vi "Open_Close.vi"(0 "VI_Reference_In":refnum<vi>, 11 "Error_In":errorcluster, 13 "Open/Close":T1=enum."Close") -> (4 "VI_Reference_Out":refnum<vi>, 15 "Error_Out":errorcluster)   [LabVIEW 2021]
doc: "Used to open and close the VI"
uses:
  Controls/Open_Close.ctl
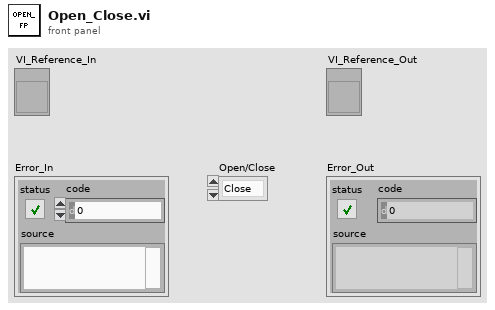
[diagram p1: front panel]
types:
  T1 = typedef "Open_Close.ctl" = enum16{"Open", "Close"}
  T2 = enum32{"Invalid", "Standard", "Closed", "Hidden", "Minimized", "Maximized"}
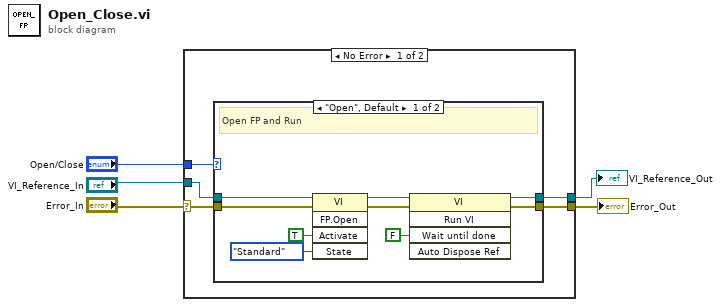
[diagram p0: block diagram]
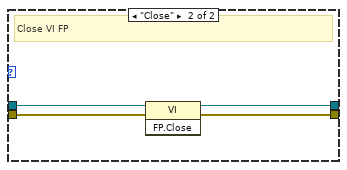
[diagram p2: hidden frame]
diagram:
  n1 = case shown="No Error" "Error_In" {
    selector: "Error_In" -> [w10 w25]
    tunnel: [w9 w25] -> w1
    tunnel: "Open/Close" -> [w8 _]
    tunnel: "VI_Reference_In" -> [w6 w24]
    tunnel: [w7 w24] -> w4
    frame No Error {
      n2 = case shown="\"Open\", Default" w8 {
        tunnel: w10 -> [w19 w22]
        tunnel: [w18 w23] -> w9
        tunnel: w6 -> [w16 w21]
        tunnel: [w14 w20] -> w7
        frame "Open", Default {
          # "Open FP and Run"
          n3 = invoke class="VI" method="FP.Open"(reference=w16, error in=w19, "Activate"=TRUE ("Activate?"), "State"=T2."Standard") -> (reference out=w15:refnum<vi>, error out=w17:errorcluster)  [unwired: 1 in, 3 out]
          n4 = invoke class="VI" method="Run VI"(reference=w15, error in=w17, "Wait until done"=FALSE ("Wait Until Done")) -> (reference out=w14:refnum<vi>, error out=w18:errorcluster)  [unwired: 2 in, 3 out]
        }
        frame "Close" {
          # "Close VI FP"
          n5 = invoke class="VI" method="FP.Close"(reference=w21, error in=w22) -> (reference out=w20:refnum<vi>, error out=w23:errorcluster)  [unwired: 1 in, 1 out]
        }
      }
    }
    frame Error {
    }
  }
  "VI_Reference_Out" <- w4
  "Error_Out" <- w1
